vi "FlatToRichniswitch_grpc_GetAttributeViStringRequest.vi"(5 "OutputClusterType":T1, 11 "InputCluster":T4) -> (3 "OutputCluster":T1)   [LabVIEW 2021, in "NI Switch_client.lvlib"]
uses:
  NI Switch_client.lvlib
  niswitch_grpc_NiSwitchAttribute.ctl
  nidevice_grpc_Session.ctl
  niswitch_grpc_GetAttributeViStringRequest.ctl
  nidevice_grpc_Session_Flat.ctl
  niswitch_grpc_GetAttributeViStringRequest_Flat.ctl
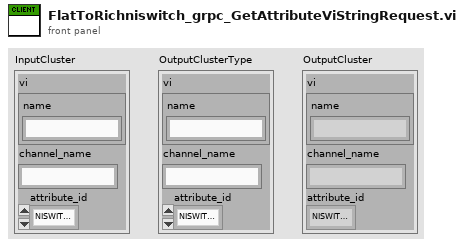
[diagram p1: front panel]
types:
  T1 = typedef "NI Switch_client.lvlib/niswitch_grpc_GetAttributeViStringRequest.ctl" = cluster{"vi":T2, "channel_name":string, "attribute_id":T3}
  T2 = typedef "NI Switch_client.lvlib/nidevice_grpc_Session.ctl" = cluster{"name":string}
  T3 = typedef "NI Switch_client.lvlib/niswitch_grpc_NiSwitchAttribute.ctl" = enum32{"NISWITCH_ATTRIBUTE_UNSPECIFIED", "NISWITCH_ATTRIBUTE_RANGE_CHECK", "NISWITCH_ATTRIBUTE_QUERY_INSTRUMENT_STATUS", "NISWITCH_ATTRIBUTE_CACHE", "NISWITCH_ATTRIBUTE_SIMULATE", "NISWITCH_ATTRIBUTE_RECORD_COERCIONS", "NISWITCH_ATTRIBUTE_DRIVER_SETUP", "NISWITCH_ATTRIBUTE_INTERCHANGE_CHECK", "NISWITCH_ATTRIBUTE_CHANNEL_COUNT", "NISWITCH_ATTRIBUTE_SPECIFIC_DRIVER_PREFIX", "NISWITCH_ATTRIBUTE_IO_RESOURCE_DESCRIPTOR", "NISWITCH_ATTRIBUTE_LOGICAL_NAME", "NISWITCH_ATTRIBUTE_SUPPORTED_INSTRUMENT_MODELS", "NISWITCH_ATTRIBUTE_GROUP_CAPABILITIES", "NISWITCH_ATTRIBUTE_INSTRUMENT_FIRMWARE_REVISION", "NISWITCH_ATTRIBUTE_INSTRUMENT_MANUFACTURER", "NISWITCH_ATTRIBUTE_INSTRUMENT_MODEL", "NISWITCH_ATTRIBUTE_SPECIFIC_DRIVER_VENDOR", "NISWITCH_ATTRIBUTE_SPECIFIC_DRIVER_DESCRIPTION", "NISWITCH_ATTRIBUTE_SPECIFIC_DRIVER_CLASS_SPEC_MAJOR_VERSION", "NISWITCH_ATTRIBUTE_SPECIFIC_DRIVER_CLASS_SPEC_MINOR_VERSION", "NISWITCH_ATTRIBUTE_SPECIFIC_DRIVER_REVISION", "NISWITCH_ATTRIBUTE_SERIAL_NUMBER_I32", "NISWITCH_ATTRIBUTE_IS_WAITING_FOR_TRIG", "NISWITCH_ATTRIBUTE_TRIGGER_MODE", "NISWITCH_ATTRIBUTE_MASTER_SLAVE_TRIGGER_BUS", "NISWITCH_ATTRIBUTE_MASTER_SLAVE_SCAN_ADVANCED_BUS", "NISWITCH_ATTRIBUTE_CABLED_MODULE_TRIGGER_BUS", "NISWITCH_ATTRIBUTE_CABLED_MODULE_SCAN_ADVANCED_BUS", "NISWITCH_ATTRIBUTE_TRIGGER_INPUT_POLARITY", "NISWITCH_ATTRIBUTE_SCAN_ADVANCED_POLARITY", "NISWITCH_ATTRIBUTE_PARSED_SCAN_LIST", "NISWITCH_ATTRIBUTE_HANDSHAKING_INITIATION", "NISWITCH_ATTRIBUTE_NUMBER_OF_RELAYS", "NISWITCH_ATTRIBUTE_SERIAL_NUMBER", "NISWITCH_ATTRIBUTE_DIGITAL_FILTER_ENABLE", "NISWITCH_ATTRIBUTE_POWER_DOWN_LATCHING_RELAYS_AFTER_DEBOUNCE", "NISWITCH_ATTRIBUTE_ANALOG_BUS_SHARING_ENABLE", "NISWITCH_ATTRIBUTE_TEMPERATURE", "NISWITCH_ATTRIBUTE_IS_SOURCE_CHANNEL", "NISWITCH_ATTRIBUTE_IS_DEBOUNCED", "NISWITCH_ATTRIBUTE_IS_CONFIGURATION_CHANNEL", "NISWITCH_ATTRIBUTE_SETTLING_TIME", "NISWITCH_ATTRIBUTE_BANDWIDTH", "NISWITCH_ATTRIBUTE_MAX_DC_VOLTAGE", "NISWITCH_ATTRIBUTE_MAX_AC_VOLTAGE", "NISWITCH_ATTRIBUTE_MAX_SWITCHING_DC_CURRENT", "NISWITCH_ATTRIBUTE_MAX_SWITCHING_AC_CURRENT", "NISWITCH_ATTRIBUTE_MAX_CARRY_DC_CURRENT", "NISWITCH_ATTRIBUTE_MAX_CARRY_AC_CURRENT", "NISWITCH_ATTRIBUTE_MAX_SWITCHING_DC_POWER", "NISWITCH_ATTRIBUTE_MAX_SWITCHING_AC_POWER", "NISWITCH_ATTRIBUTE_MAX_CARRY_DC_POWER", "NISWITCH_ATTRIBUTE_MAX_CARRY_AC_POWER", "NISWITCH_ATTRIBUTE_CHARACTERISTIC_IMPEDANCE", "NISWITCH_ATTRIBUTE_WIRE_MODE", "NISWITCH_ATTRIBUTE_NUM_OF_ROWS", "NISWITCH_ATTRIBUTE_NUM_OF_COLUMNS", "NISWITCH_ATTRIBUTE_SCAN_LIST", "NISWITCH_ATTRIBUTE_SCAN_MODE", "NISWITCH_ATTRIBUTE_TRIGGER_INPUT", "NISWITCH_ATTRIBUTE_SCAN_ADVANCED_OUTPUT", "NISWITCH_ATTRIBUTE_IS_SCANNING", "NISWITCH_ATTRIBUTE_SCAN_DELAY", "NISWITCH_ATTRIBUTE_CONTINUOUS_SCAN"}
  T4 = typedef "NI Switch_client.lvlib/niswitch_grpc_GetAttributeViStringRequest_Flat.ctl" = cluster{"vi":T5, "channel_name":string, "attribute_id":T3}
  T5 = typedef "NI Switch_client.lvlib/nidevice_grpc_Session_Flat.ctl" = cluster{"name":string}
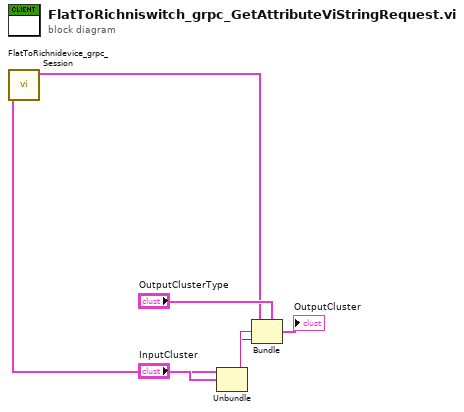
[diagram p0: block diagram]
diagram:
  n1 = Unbundle "Unbundle"("InputCluster") -> ("vi"=w4:T5, "channel_name"=w2:string, "attribute_id"=w1:T3)
  n2 = call "FlatToRichnidevice_grpc_Session.vi"("InputCluster"=w4) -> ("OutputCluster"=w3:T2)  [unwired: 10 in]
  n3 = Bundle "Bundle"(cluster="OutputClusterType", "vi"=w3, "channel_name"=w2, "attribute_id"=w1) -> (→"OutputCluster":T1)
